vi "Serial Port - Find used serial ports.vi"(8 "error in (no error)":errorcluster, 9 "Selected Values":string[](array[string]), 10 "COM Ports list":string[](array[string])) -> (0 "error out":errorcluster, 3 "Items to disable":i32[](array[numeric]))   [LabVIEW 2011]
doc: "Creates a list with a numeric representation of the selected COM ports. If a COM port is selected, it should be disabled in all other controls."
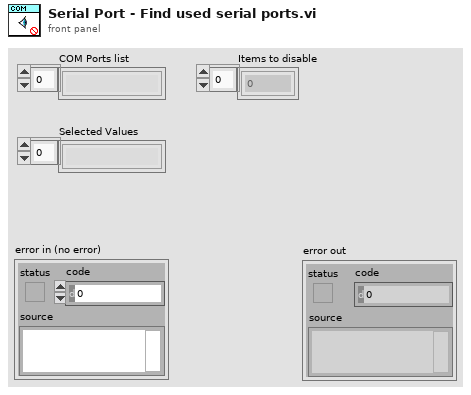
[diagram p1: front panel]
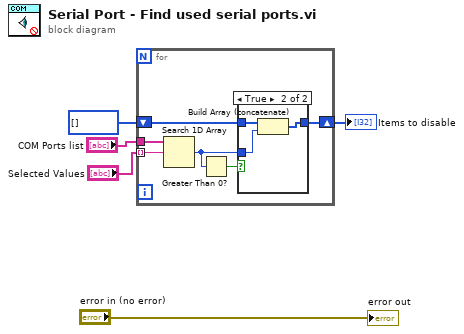
[diagram p0: block diagram]
diagram:
  n1 = for {
    tunnel: "Selected Values" -> [w6] mode=indexing
    tunnel: "COM Ports list" -> [w11]
    shift-right: [w9] -> w5
    shift-left: i32[] [] -> [w8]
    n2 = Search 1D Array(1D array=w11, element=w6) -> (index of element=w7:i32)  [unwired: 1 in]
    n3 = Greater Than 0?(x=w7) -> (x > 0?=w10:bool)
    n4 = case shown="True" w10 {
      tunnel: w7 -> [_ w15]
      tunnel: [w12 w14] -> w9
      tunnel: w8 -> [w12 w13]
      frame False {
      }
      frame True {
        n5 = Build Array (concatenate)(w13, w15) -> (w14:i32[])
      }
    }
  }
  "Items to disable" <- w5
  "error out" <- "error in (no error)"
